vi "Process Data.vi"(8 "error in":errorcluster, 11 "Example Plugin in":refnum<class "Example Plugin.lvclass">) -> (0 "error out":errorcluster, 3 "Example Plugin out":refnum<class "Example Plugin.lvclass">)   [LabVIEW 2023, in "Example Plugin.lvclass"]
uses:
  Example Plugin.lvclass
  Example Plugin.lvclass/Example Plugin.ctl
  Capabilities/Voltage/Voltage Control.lvclass
  Capabilities/Voltage/Read Voltage Setpoint (Single).vi
  Capabilities/Cycler/Cycler.lvclass
  Capabilities/Current/Current Control.lvclass
  Capabilities/Current/Read Current Setpoint (Single).vi
panel:
  out "Current Setpoint":dbl
  out "Voltage Setpoint":dbl
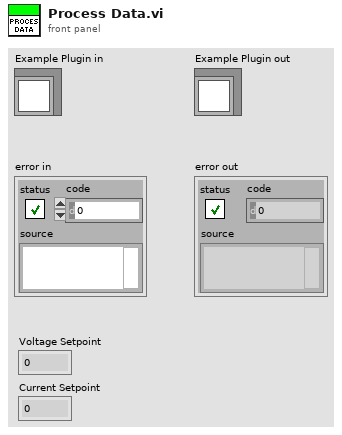
[diagram p1: front panel]
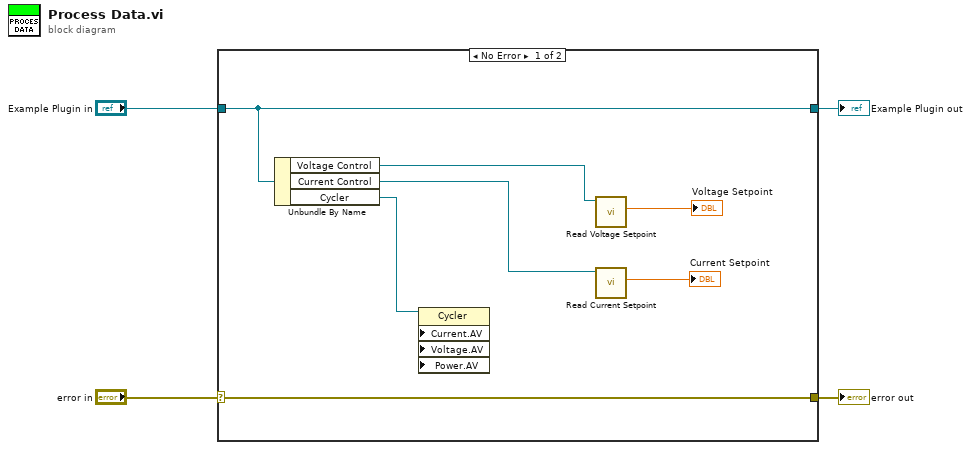
[diagram p0: block diagram]
diagram:
  n1 = case shown="No Error" "error in" {
    selector: "error in" -> [w5 w13]
    tunnel: [w5 w13] -> w3
    tunnel: [w11 w12] -> w1
    tunnel: "Example Plugin in" -> [w11 w12]
    frame No Error {
      n2 = Unbundle By Name(w11) -> ("Voltage Control"=w7:refnum<class "Voltage Control.lvclass">, "Current Control"=w8:refnum<class "Current Control.lvclass">, "Cycler"=w10:refnum<class "Cycler.lvclass">)
      n3 = property class="Cycler" props=["Current.AV", "Voltage.AV", "Power.AV"](reference=w10) -> ()  [unwired: 4 in, 2 out]
      n4 = call-poly "Read Voltage Setpoint.vi"("Voltage Control in"=w7) -> ("Voltage Setpoint"=→"Voltage Setpoint":dbl)  [unwired: 7 in, 3 out]
      n5 = call-poly "Read Current Setpoint.vi"("Current Control in"=w8) -> ("Current Setpoint"=→"Current Setpoint":dbl)  [unwired: 7 in, 3 out]
    }
    frame Error {
    }
  }
  "error out" <- w3
  "Example Plugin out" <- w1
